vi "Pick RPS Play.vi"(10 "Result":T2, 11 "Them":T1) -> (3 "You":T1)   [LabVIEW 2022 SP3, in "AoC22.lvlib"]
uses:
  AoC22.lvlib
  RPS Play.ctl
  RPS Result.ctl
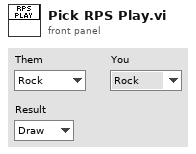
[diagram p1: front panel]
types:
  T1 = typedef "AoC22.lvlib/RPS Play.ctl" = enum16{"Rock", "Paper", "Scissors"}
  T2 = typedef "AoC22.lvlib/RPS Result.ctl" = enum16{"Draw", "Win", "Lose"}
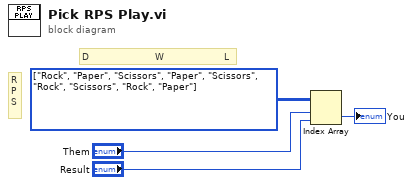
[diagram p0: block diagram]
diagram:
  w4 = T1[][] [[enum."Rock", enum."Paper", enum."Scissors"], [enum."Paper", enum."Scissors", enum."Rock"], [enum."Scissors", enum."Rock", enum."Paper"]] items=["Rock", "Paper", "Scissors"]
  # "D                      W                    L"
  # "R\nP\nS"
  n1 = Index Array(array=w4, index (row)="Them", index (col)="Result") -> (element=→"You":T1)
